vi "GetMessageLength.vi"(8 "error in (no error)":errorcluster, 11 "TCP_Client in":refnum<class "TCP_Client.lvclass">) -> (0 "error out":errorcluster, 3 "TCP_Client out":refnum<class "TCP_Client.lvclass">)   [LabVIEW 2023, in "TCP_Client.lvlib" / "TCP_Client.lvclass"]
uses:
  TCP_Client.lvclass
  C:/Program Files (x86)/National Instruments/LabVIEW 2023/vi.lib/ActorFramework/Actor/Actor.lvclass
  <vilib>/ActorFramework/Actor/Actor.lvclass/Actor.ctl
  <vilib>/ActorFramework/Message Enqueuer/Message Enqueuer.lvclass/Message Enqueuer.ctl
  TCP_Client.lvclass/TCP_Client.ctl
  TCP_Client Messages/DisabelConnectButton Msg/DisabelConnectButton Msg.lvclass/DisabelConnectButton Msg.ctl
  <vilib>/ActorFramework/Message Enqueuer/Init from Existing Queue.vi
  <vilib>/ActorFramework/Message Enqueuer/Enqueue.vi
  TCP_Client Messages/LookForStartOfMessage Msg/LookForStartOfMessage Msg.lvclass
  C:/Program Files (x86)/National Instruments/LabVIEW 2023/vi.lib/ActorFramework/Message/Message.lvclass
  TCP_Client Messages/DisabelConnectButton Msg/DisabelConnectButton Msg.lvclass
  <vilib>/ActorFramework/Message Priority Queue/Priority Enqueue.vi
  <vilib>/ActorFramework/Message Enqueuer/Message Enqueuer.lvclass
  <vilib>/ActorFramework/Actor/Actor.lvclass
  TCP_Client Messages/ReadMessage Msg/ReadMessage Msg.lvclass
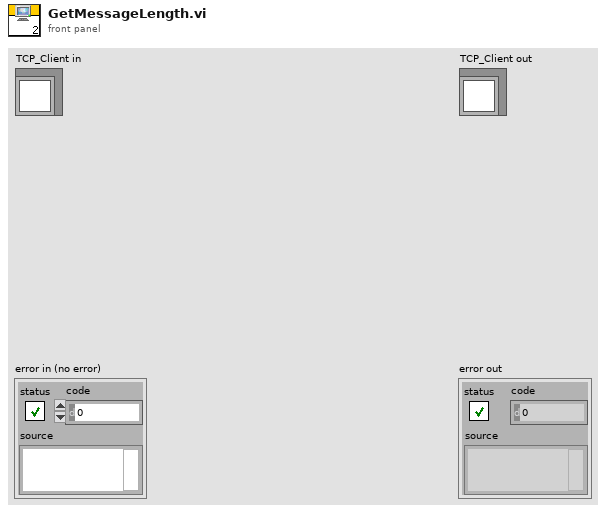
[diagram p1: front panel]
types:
  T1 = enum8{"Enabled", "Disabled", "Disabled and Grayed Out"}
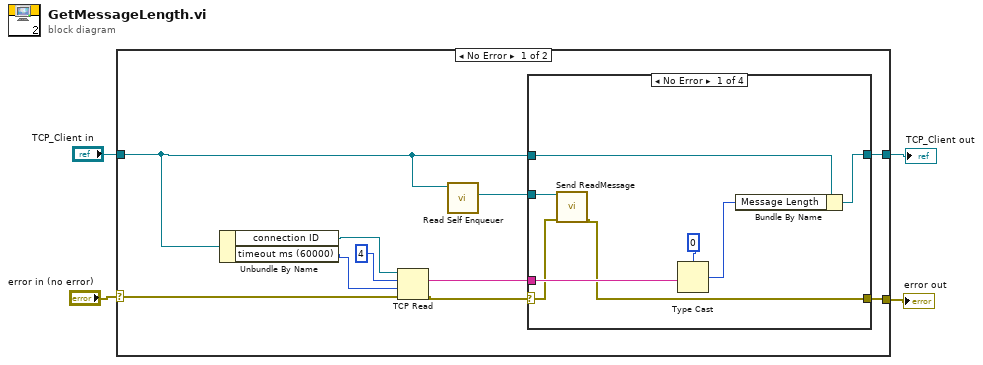
[diagram p0: block diagram]
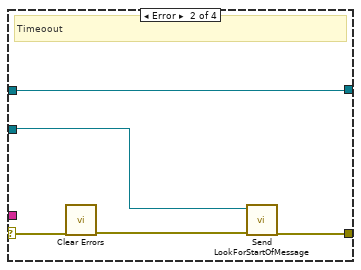
[diagram p2: hidden frame]
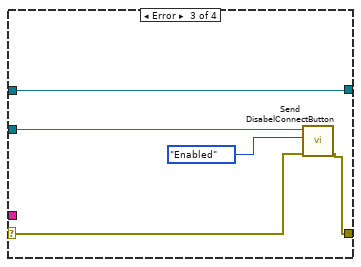
[diagram p3: hidden frame]
diagram:
  n1 = case shown="No Error" "error in (no error)" {
    selector: "error in (no error)" -> [w5 w36]
    tunnel: [w6 w36] -> w3
    tunnel: [w9 w35] -> w1
    tunnel: "TCP_Client in" -> [w8 w35]
    frame No Error {
      n2 = Unbundle By Name(w8) -> ("connection ID"=w14:refnum<k5>, "timeout ms (60000)"=w12:i32)
      n3 = TCP Read(connection ID=w14, bytes to read=4, error in (no error)=w5, 9:w12) -> (data out=w10:string, error out=w11:errorcluster)  [unwired: 1 in, 1 out]
      n4 = call <vilib>:"Read Self Enqueuer.vi"("Actor"=w8) -> ("Self Enqueuer"=w7:refnum<class "Message Enqueuer.lvclass">)  [unwired: 10 in]
      n5 = case shown="No Error" w11 {
        selector: w11 -> [w16 w26 w30 w34]
        tunnel: w10 -> [w22 _ _ _]
        tunnel: w8 -> [w20 w27 w28 w33]
        tunnel: [w18 w27 w28 w33] -> w9
        tunnel: w7 -> [w17 w25 w32 _]
        tunnel: [w15 w23 w29 w34] -> w6
        frame No Error {
          n6 = call "Send ReadMessage.vi"("error in (no error)"=w16, "Message Enqueuer"=w17) -> ("error out"=w15:errorcluster)  [unwired: 8 in, 1 out]
          n7 = Type Cast(type=0, x=w22) -> (*(type *) &x=w19:i32)
          n8 = Bundle By Name(cluster=w20, "Message Length"=w19) -> (w18:refnum<class "TCP_Client.lvclass">)
        }
        frame Error {
          # "Timeoout"
          n9 = call <vilib>:"Clear Errors.vi"("error in (no error)"=w26) -> ("error out"=w24:errorcluster)  [unwired: 5 in, 1 out]
          n10 = call "Send LookForStartOfMessage.vi"("error in (no error)"=w24, "Message Enqueuer"=w25) -> ("error out"=w23:errorcluster)  [unwired: 8 in, 1 out]
        }
        frame Error {
          n11 = call "Send DisabelConnectButton.vi"("error in (no error)"=w30, "Connect button Disabled"=T1."Enabled", "Message Enqueuer"=w32) -> ("error out"=w29:errorcluster)  [unwired: 7 in, 1 out]
        }
        frame Default {
        }
      }
    }
    frame Error {
    }
  }
  "error out" <- w3
  "TCP_Client out" <- w1
